vi "M_TestDataFGV.vi"(6 "DataFilePath":path, 7 "TestFgvCMD":T3, 9 "Status":T1, 10 "OK?":bool, 11 "TestData In":T2) -> (3 "TestData Out":T2)   [LabVIEW 2021]
uses:
  TestFgvCMD.ctl
  TcpCmd_003/SubVI/TestMeasurementStatus.ctl
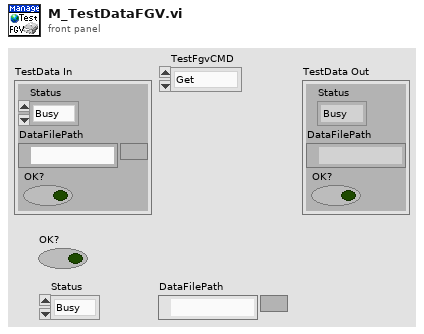
[diagram p1: front panel]
types:
  T1 = typedef "TestMeasurementStatus.ctl" = enum16{"Busy", "Ready", "Done", "Error"}
  T2 = cluster{"Status":T1, "DataFilePath":path, "OK?":bool}
  T3 = typedef "TestFgvCMD.ctl" = enum16{"Get", "Set", "SetOK?", "SetStatus", "SetDataPath"}
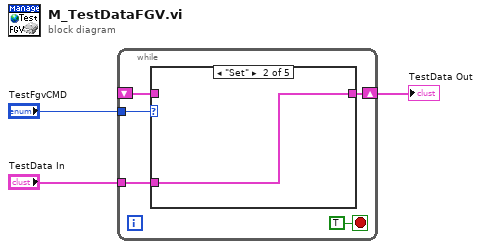
[diagram p0: block diagram]
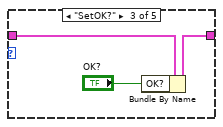
[diagram p3: hidden frame]
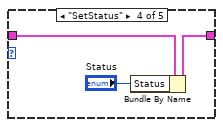
[diagram p4: hidden frame]
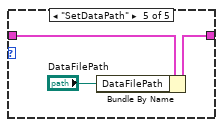
[diagram p5: hidden frame]
diagram:
  n1 = while {
    tunnel: "TestData In" -> [w5]
    tunnel: "TestFgvCMD" -> [w7]
    shift-right: [w6] -> w1
    shift-left: _ -> [w4]
    stop <- TRUE stop-if-true
    n2 = case shown="\"Set\"" w7 {
      tunnel: [w9 w10 w12 w15 w18] -> w6
      tunnel: w5 -> [_ w10 _ _ _]
      tunnel: w4 -> [w9 _ w13 w16 w19]
      frame "Get", Default {
      }
      frame "Set" {
      }
      frame "SetOK?" {
        n3 = Bundle By Name(cluster=w13, "OK?"="OK?") -> (w12:T2)
      }
      frame "SetStatus" {
        n4 = Bundle By Name(cluster=w16, "Status"="Status") -> (w15:T2)
      }
      frame "SetDataPath" {
        n5 = Bundle By Name(cluster=w19, "DataFilePath"="DataFilePath") -> (w18:T2)
      }
    }
  }
  "TestData Out" <- w1
